vi "Main Pressure Sensor.vi"() -> ()   [LabVIEW 2018]
uses:
  <vilib>/nisyscfg/Filter Mode.ctl
  <vilib>/Platform/TimedLoop/XDataNode/timing_clust.ctl
  <vilib>/Platform/TimedLoop/XDataNode/nitl_modes.ctl
  <vilib>/Platform/TimedLoop/XDataNode/wakeup.ctl
  <vilib>/DAQmx/read.llb/DAQmx Read (Analog DBL 1Chan 1Samp).vi
  <vilib>/DAQmx/write.llb/DAQmx Write (Analog DBL 1Chan 1Samp).vi
  <vilib>/DAQmx/create/scale.llb/DAQmx Create Scale (Linear).vi
  <vilib>/DAQmx/create/channels.llb/DAQmx Create Channel (AO-Voltage-Basic).vi
  <vilib>/DAQmx/create/channels.llb/DAQmx Create Channel (AI-Voltage-Basic).vi
  <vilib>/DAQmx/miscellaneous.llb/DAQmx Fill In Error Info.vi
  <vilib>/platform/TimedLoop/XDataNode/XDataNode.xnode
  <vilib>/nisyscfg/nisyscfg.lvlib
  <resource>/objmgr/nicriosae.rc
  <vilib>/Platform/TimedLoop/XDataNode/XDNodeRunTimeDep.lvlib
  <resource>/objmgr/daqmx.rc
panel:
  out "Voltage":dbl format="%0.2f"
  in  "Scale":dbl=3.0
  out "error out":errorcluster
  in  "Power":bool
  in  "dt (ms)":i64=1000
  out "Current File Size (kB)":dbl
  out "File Location":path
  in  "save":bool=TRUE
  out "Configuration Complete?":bool
  out "Acquisition Time":timestamp format="%<%H:%M:%S%2u>T"
  out "Pressure":dbl(graph)
  # "The code will take the input voltage and\nscale it according to the Scale value to the\nright.  The measurement is set for 0-5 V, so\nif the range of the transducer is 0-15 PSI, \nthe scale should be 3; if 0-50 PSI, it should \nbe 10.\nThe system will convert PSI to inHg using \nthe conversion of 2.03602045718904 inHg \nto 1 PSI.\nTo get the maximum resolution of the \nmeasurement, divide 10 V by the \ncard resolution (2^16 if 16 bits, 2^24 if \n24 bits).  This will give you a resolution in\nV."
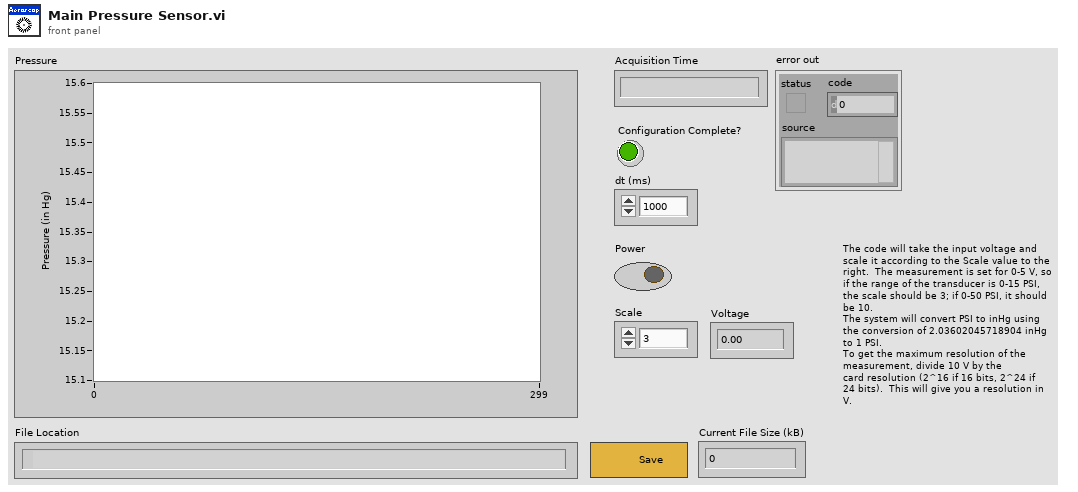
[diagram p1: front panel]
types:
  T1 = typedef "nisyscfg.lvlib/Filter Mode.ctl" = i32
  T2 = cluster{"seconds since 1Jan1904":timestamp, "data":dbl, "data 2":dbl}
  T3 = typedef "XDNodeRunTimeDep.lvlib/timing_clust.ctl" = cluster{"Expected End [f-1]":u64, "Actual End [f-1]":u64, "Finished Late? [f-1]":bool, "Expected End [i-1]":u64, "Actual End [i-1]":u64, "Finished Late? [i-1]":bool, "Expected Start [i]":u64, "Actual Start [i]":u64, "Expected Start [f]":u64, "Actual Start [f]":u64, "Source Name":string, "Structure Name":string, "Period":i64, "Deadline":i64, "Offset":i64, "Start":i64, "Priority":i32, "Timeout":i32, "Mode":T4, "Wakeup Reason":T5, "Error":errorcluster, "Source Type":string, "Secondary Source Type":string, "Global End Time":u64, "Global Start Time":u64, "Frame Duration":u64, "Iteration Duration":u64, "Assigned CPU":i32, "I/O Scan Engine Mode":u32}
  T4 = typedef "XDNodeRunTimeDep.lvlib/nitl_modes.ctl" = enum32{"No Change", "Process missed periods, maintain original phase", "Discard missed periods, maintain original phase", "Process missed periods, ignore original phase", "Discard missed periods, ignore original phase"}
  T5 = typedef "XDNodeRunTimeDep.lvlib/wakeup.ctl" = enum32{"Normal", "Aborted", "Asynchronous wakeup", "Timing source error", "Timed loop error", "Timeout"}
  T6 = cluster{"seconds since 1Jan1904":timestamp, "data":dbl, dbl}
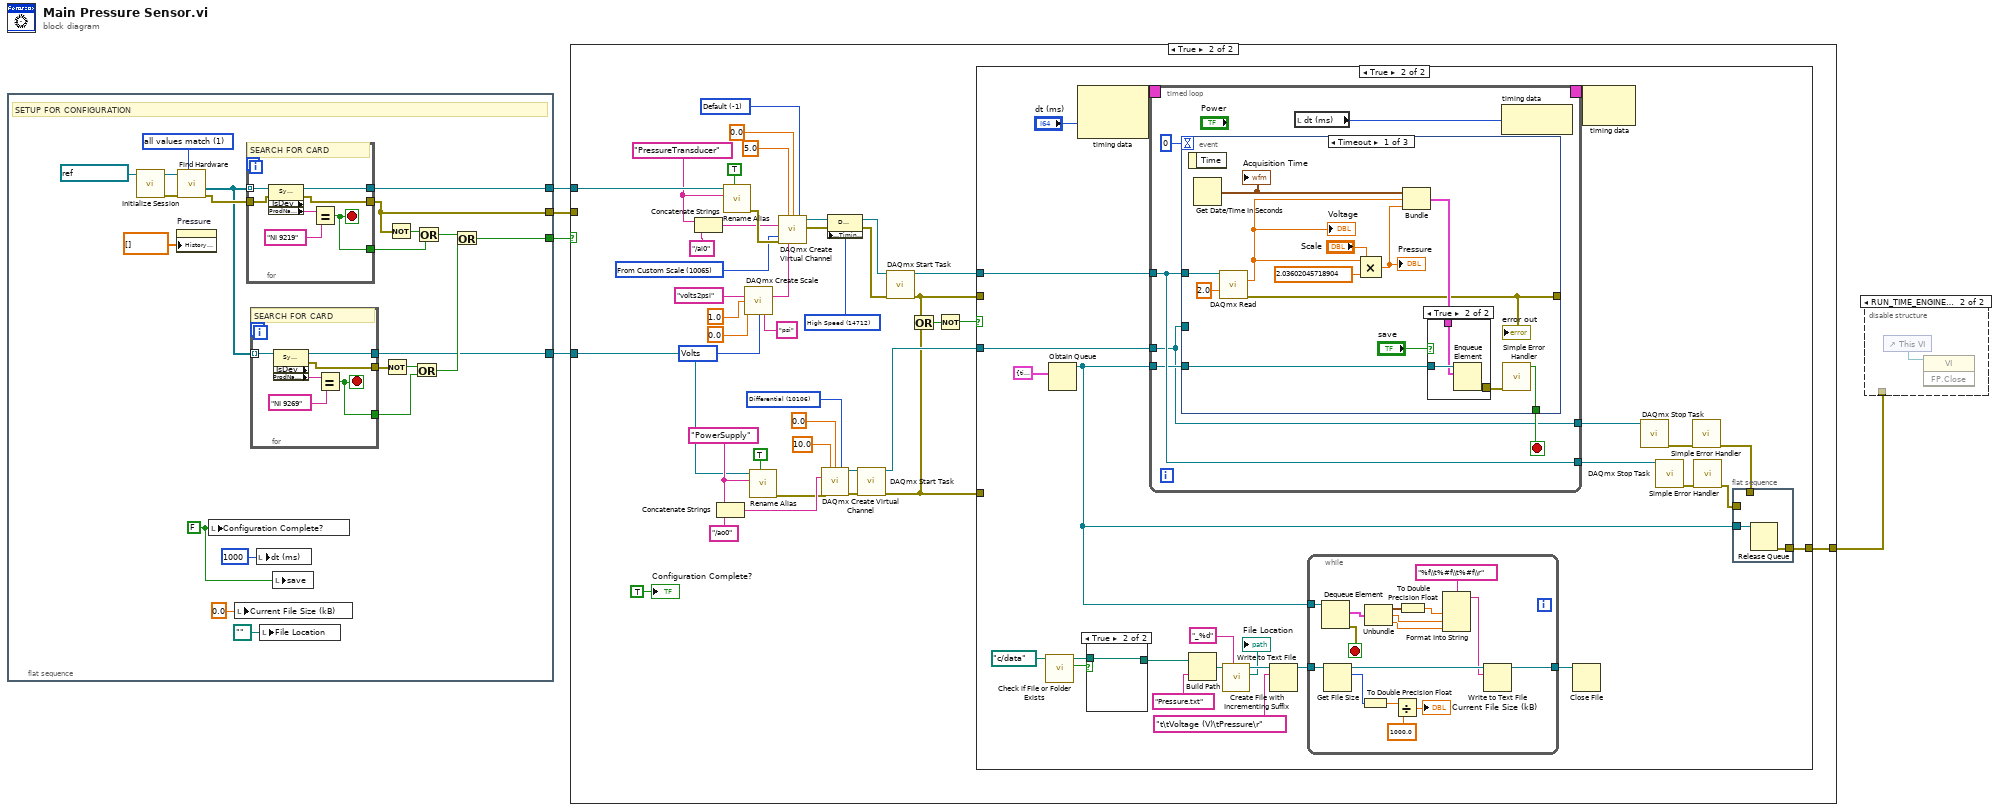
[diagram p0: block diagram]
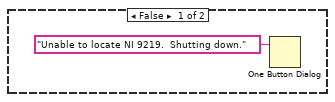
[diagram p3: hidden frame]
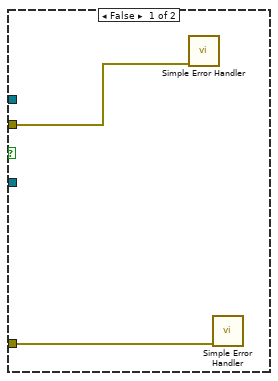
[diagram p4: hidden frame]
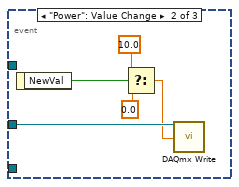
[diagram p6: hidden frame]
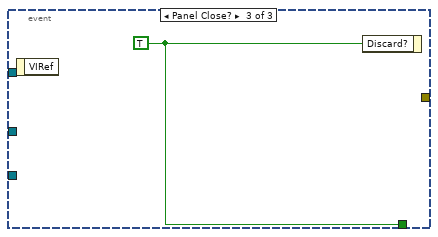
[diagram p7: hidden frame]
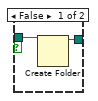
[diagram p8: hidden frame]
diagram:
  n1 = flat-sequence {
    tunnel: [w23] -> w5
    tunnel: [w20] -> w4
    tunnel: [w7] -> w3
    tunnel: [w6] -> w1
    frame #0 {
      w17 = FALSE ("Configuration Complete?")
      w24 = T1 1 items=["all values match"=1, "any value matches"=2, "values do not match"=3, "all properties exist"=4] ("Filter Mode (all values match)")
      # "SETUP FOR CONFIGURATION"
      n2 = call <vilib>:"Initialize Session.vi"("Target (localhost)"=refnum<k21> "localhost") -> ("error out"=w26:errorcluster, "Session out"=w25:refnum<k21>)  [unwired: 9 in]
      n3 = property on="Pressure" class="WFChart (strict)"("History Data"=dbl[] []) -> ()  [unwired: 2 in, 2 out]
      n4 = call <vilib>:"Find Hardware.vi"("Filter Mode (all values match)"=w24, "error in (no error)"=w26, "Session in"=w25) -> ("error out"=w22:errorcluster, "Resources out"=w13:refnum<k20>[])  [unwired: 5 in, 2 out]
      n5 = local write "Configuration Complete?"(w17) -> ()
      n6 = local write "Current File Size (kB)"(0.0 ("Current File Size (kB)")) -> ()
      n7 = for {
        tunnel: w13 -> [w40] mode=indexing
        tunnel: [w38] -> w23
        tunnel: [w37] -> w21
        tunnel: w22 -> [w36]
        tunnel: [w35] -> w20
        stop <- w37 stop-if-true
        # "SEARCH FOR CARD"
        n8 = property class="System Hardware" props=["IsDev", "ProdName"](reference=w40, error in=w36) -> (reference out=w38:refnum<k20>, error out=w35:errorcluster, "ProdName"=w34:string)  [unwired: 1 out]
        n9 = Equal?(x=w34, y="NI 9219") -> (x = y?=w37:bool)
      }
      n10 = for {
        tunnel: w13 -> [w33] mode=indexing
        tunnel: [w31] -> w6
        tunnel: [w30] -> w10
        tunnel: [w29] -> w12
        stop <- w30 stop-if-true
        # "SEARCH FOR CARD"
        n11 = property class="System Hardware" props=["IsDev", "ProdName"](reference=w33) -> (reference out=w31:refnum<k20>, error out=w29:errorcluster, "ProdName"=w28:string)  [unwired: 1 in, 1 out]
        n12 = Equal?(x=w28, y="NI 9269") -> (x = y?=w30:bool)
      }
      n13 = local write "dt (ms)"(i64 1000 ("dt (ms)")) -> ()
      n14 = local write "File Location"(path "" ("File Location")) -> ()
      n15 = local write "save"(w17) -> ()
      n16 = Not(x=w12) -> (.not. x?=w11:bool)
      n17 = Not(x=w20) -> (.not. x?=w19:bool)
      n18 = Or(x=w11, y=w10) -> (x .or. y?=w9:bool)
      n19 = Or(x=w19, y=w21) -> (x .or. y?=w8:bool)
      n20 = Or(x=w8, y=w9) -> (x .or. y?=w7:bool)
    }
  }
  n21 = case shown="True" w3 {
    tunnel: w4 -> [_ _]
    tunnel: w5 -> [_ w80]
    tunnel: [_ w76] -> w2
    tunnel: w1 -> [_ w59]
    frame False {
      n22 = One Button Dialog(message="Unable to locate NI 9219.  Shutting down.") -> ()  [unwired: 1 in, 1 out]
    }
    frame True {
      w46 = 14712 items=["High Resolution"=10195, "High Speed"=14712, "Best 50 Hz Rejection"=14713, "Best 60 Hz Rejection"=14714, "Custom"=10137] ("AI.ADCTimingMode")
      w53 = 10106 items=["Default"=-1, "RSE"=10083, "Differential"=10106, "Pseudodifferential"=12529] ("output terminal configuration")
      w62 = "PowerSupply" ("New Name")
      w66 = 10348 items=["Volts"=10348, "Amps"=10342, "Deg F"=10144, "Deg C"=10143, "Deg R"=10145, "Kelvins"=10325, "Strain"=10299, "Ohms"=10384, "Hz"=10373, "Seconds"=10364, "Meters"=10219, "Inches"=10379, "Degrees"=10146, "Radians"=10273, "Ticks"=10304, "g"=10186, "m/s^2"=12470, "m/s"=15959, "in/s"=15960, "Pascals"=10081, "Newtons"=15875, "Pounds"=15876, "kgf"=15877, "psi"=15879, "bar"=15880, "Nm"=15881, "oz-in"=15882, "lb-in"=15883, "lb-ft"=15884, "Volts/Volt"=15896, "mVolts/Volt"=15897, "pCoulombs"=16103, "Coulombs"=16102, "From TEDS"=12516] ("pre-scaled units")
      w69 = 10065 items=["Volts"=10348, "From Custom Scale"=10065] ("units")
      w72 = -1 items=["Default"=-1, "RSE"=10083, "NRSE"=10078, "Differential"=10106, "Pseudodifferential"=12529] ("input terminal configuration")
      w75 = "PressureTransducer" ("New Name")
      n23 = Concatenate Strings(w75, "/ai0" ("string")) -> (w73:string)
      n24 = Concatenate Strings(w62, "/ao0" ("string")) -> (w57:string)
      n25 = call <vilib>:"Rename Alias.vi"("Update Dependencies (T)"=TRUE, "New Name"=w75, "Resource in"=w80) -> ("error out"=w74:errorcluster)  [unwired: 5 in, 3 out]
      n26 = call-poly <vilib>:"DAQmx Create Scale.vi"("name"="volts2psi", "slope"=1.0, "y-intercept"=0.0, "pre-scaled units"=w66, "scaled units"="psi") -> ("scale out"=w64:tag)  [unwired: 9 in, 1 out]
      n27 = call <vilib>:"Rename Alias.vi"("Update Dependencies (T)"=TRUE, "New Name"=w62, "Resource in"=w59) -> ("error out"=w47:errorcluster)  [unwired: 5 in, 3 out]
      n28 = call-poly <vilib>:"DAQmx Create Virtual Channel.vi"("maximum value"=5.0, "minimum value"=0.0, "input terminal configuration"=w72, "physical channels"=w73, "units"=w69, "error in"=w74, "custom scale name"=w64) -> ("task out"=w45:refnum<k21>, "error out"=w43:errorcluster)  [unwired: 7 in]
      n29 = call-poly <vilib>:"DAQmx Create Virtual Channel.vi"("maximum value"=10.0, "minimum value"=0.0, "output terminal configuration"=w53, "physical channels"=w57, "error in"=w47) -> ("task out"=w56:refnum<k21>, "error out"=w58:errorcluster)  [unwired: 9 in]
      n30 = property class="DAQmx Channel"(reference=w45, error in=w43, "Analog Input:General Properties:Digitizer/ADC:Timing Mode"=w46) -> (reference out=w44:refnum<k21>, error out=w42:errorcluster)
      n31 = call <vilib>:"DAQmx Start Task.vi"("task/channels in"=w56, "error in"=w58) -> ("task out"=w52:refnum<k21>, "error out"=w48:errorcluster)  [unwired: 12 in]
      n32 = call <vilib>:"DAQmx Start Task.vi"("task/channels in"=w44, "error in"=w42) -> ("task out"=w77:refnum<k21>, "error out"=w49:errorcluster)  [unwired: 12 in]
      n33 = Or(x=w49, y=w48) -> (x .or. y?=w51:bool)
      n34 = Not(x=w51) -> (.not. x?=w50:bool)
      n35 = case shown="True" w50 {
        tunnel: w77 -> [_ w109]
        tunnel: [_ w92] -> w76
        tunnel: w52 -> [_ w87]
        tunnel: w49 -> [w83 _]
        tunnel: w48 -> [w82 _]
        frame False {
          n36 = call <vilib>:"Simple Error Handler.vi"("error in (no error)"=w83) -> ()  [unwired: 4 in, 5 out]
          n37 = call <vilib>:"Simple Error Handler.vi"("error in (no error)"=w82) -> ()  [unwired: 4 in, 5 out]
        }
        frame True {
          n38 = call <vilib>:"Check if File or Folder Exists.vi"("path"=path "c:/data") -> ("file or folder exists?"=w103:bool, "dup path"=w102:path)  [unwired: 8 in, 1 out]
          n39 = Obtain Queue(element data type=T2 {"seconds since 1Jan1904"=timestamp(0 s since 1904-01-01), "data"=0.0, "data 2"=0.0} ("output cluster")) -> (queue out=w106:refnum<queue>)  [unwired: 4 in, 2 out]
          n40 = node-c288("dt (ms)") -> (w90:T3)  [unwired: 1 in]
          n41 = case shown="True" w103 {
            tunnel: w102 -> [w147 w148]
            tunnel: [w146 w148] -> w101
            frame False {
              n42 = Create Folder(path (use dialog)=w147) -> (created path=w146:path)  [unwired: 2 in, 2 out]
            }
            frame True {
            }
          }
          n43 = timed-loop {
            tunnel: w109 -> [w113]
            tunnel: [w113] -> w108
            tunnel: w106 -> [w112]
            timing: w90 -> [_]
            timing-out: [_] -> w89
            tunnel: w87 -> [w110]
            tunnel: [w110] -> w86
            stop <- w115 stop-if-true
            n44 = event shown="[0] Timeout" {
              selector: _ -> [_ _ _]
              dyn-events: _ -> [_ _ _]
              timeout: 0 -> [_ _ _]
              tunnel: [w131 _ w140] -> w115
              tunnel: w113 -> [w127 _ _]
              tunnel: w112 -> [w130 _ _]
              tunnel: w110 -> [_ w139 _]
              tunnel: [w124 _ _] -> _
              event Timeout {
                n45 = event-data() -> ()  [unwired: 1 in, 1 out]
                n46 = Get Date/Time In Seconds() -> (seconds since 1Jan1904=w126:timestamp)
                "Acquisition Time" <- w126
                n47 = call-poly <vilib>:"DAQmx Read.vi"("task/channels in"=w127, "timeout"=2.0) -> ("data"=w119:dbl, "error out"=w124:errorcluster)  [unwired: 11 in, 1 out]
                "error out" <- w124
                "Voltage" <- w119
                n48 = Compound Arithmetic op=MULTIPLY(w119, "Scale", 2.03602045718904 ("value")) -> (w122:dbl)
                "Pressure" <- w122
                n49 = Bundle("seconds since 1Jan1904"=w126, "data"=w119, w122) -> (w125:T6)  [unwired: 1 in]
                n50 = case shown="True" "save" {
                  tunnel: w130 -> [_ w134]
                  tunnel: [_ w133] -> w128
                  tunnel: w125 -> [_ w132]
                  frame False {
                  }
                  frame True {
                    n51 = Enqueue Element(queue=w134, element=w132) -> (error out=w133:errorcluster)  [unwired: 2 in, 2 out]
                  }
                }
                n52 = call <vilib>:"Simple Error Handler.vi"("error in (no error)"=w128) -> ("error?"=w131:bool)  [unwired: 4 in, 4 out]
              }
              event "Power": Value Change {
                n53 = event-data() -> ("NewVal"=w138:bool)  [unwired: 1 in]
                n54 = Select(t=10.0, s=w138, f=0.0) -> (s? t:f=w135:dbl)
                n55 = call-poly <vilib>:"DAQmx Write.vi"("task/channels in"=w139, "data"=w135) -> ()  [unwired: 11 in, 3 out]
              }
              event Panel Close? {
                w140 = TRUE
                n56 = event-data() -> ()  [unwired: 1 in, 1 out]
                n57 = event-data("Discard?"=w140) -> ()  [unwired: 1 in, 1 out]
              }
            }
            n58 = local read "dt (ms)"() -> (w111:i64)
            n59 = node-c288(w111) -> ()  [unwired: 1 out]
          }
          n60 = Build Path(base path=w101, name or relative path="Pressure.txt") -> (appended path=w94:path)
          n61 = call <vilib>:"Create File with Incrementing Suffix.vi"("format string (\" (%d)\")"="_%d" ("format string (\" (%d)\")"), "file path"=w94) -> ("actual path"=→"File Location":path, "refnum out"=w96:refnum<file>)  [unwired: 7 in, 1 out]
          n62 = Write to Text File(file (use dialog)=w96, text="t\tVoltage (V)\tPressure\r") -> (refnum out=w95:refnum<file>)  [unwired: 2 in, 2 out]
          n63 = while {
            tunnel: w106 -> [w166]
            tunnel: w95 -> [w161]
            tunnel: [w164] -> w98
            stop <- w165 stop-if-true
            n64 = Dequeue Element(queue=w166) -> (element=w157:T2, error out=w165:errorcluster)  [unwired: 2 in, 2 out]
            n65 = Get File Size(file=w161) -> (refnum out=w160:refnum<file>, size (in bytes)=w159:i64)  [unwired: 1 in, 1 out]
            n66 = To Double Precision Float(number=w159) -> (double precision float=w158:dbl)
            n67 = Unbundle(w157) -> ("seconds since 1Jan1904"=w156:timestamp, "data"=w153:dbl, "data 2"=w151:dbl)
            n68 = Divide(x=w158, y=1000.0) -> (x/y=→"Current File Size (kB)":dbl)
            n69 = To Double Precision Float(number=w156) -> (double precision float=w154:dbl)
            n70 = Format Into String(format string="%f\\t%#f\\t%#f\\r", w154, w153, w151) -> (resulting string=w152:string)  [unwired: 2 in, 1 out]
            n71 = Write to Text File(file (use dialog)=w160, text=w152) -> (refnum out=w164:refnum<file>)  [unwired: 2 in, 2 out]
          }
          n72 = Close File(refnum=w98) -> ()  [unwired: 1 in, 2 out]
          n73 = node-c288(w89) -> ()  [unwired: 1 out]
          n74 = call <vilib>:"DAQmx Stop Task.vi"("task/channels in"=w86) -> ("error out"=w85:errorcluster)  [unwired: 13 in, 1 out]
          n75 = call <vilib>:"DAQmx Stop Task.vi"("task/channels in"=w108) -> ("error out"=w107:errorcluster)  [unwired: 13 in, 1 out]
          n76 = call <vilib>:"Simple Error Handler.vi"("error in (no error)"=w85) -> ("error out"=w84:errorcluster)  [unwired: 4 in, 4 out]
          n77 = call <vilib>:"Simple Error Handler.vi"("error in (no error)"=w107) -> ("error out"=w105:errorcluster)  [unwired: 4 in, 4 out]
          n78 = flat-sequence {
            tunnel: w106 -> [w150]
            tunnel: w105 -> [_]
            tunnel: [w149] -> w92
            tunnel: w84 -> [_]
            frame #0 {
              n79 = Release Queue(queue=w150) -> (error out=w149:errorcluster)  [unwired: 2 in, 2 out]
            }
          }
        }
      }
      "Configuration Complete?" <- TRUE ("Configuration Complete?")
    }
  }
  n80 = disable-structure shown="RUN_TIME_ENGINE==True" {
    disable-tunnel: w2 -> [_ _]
    frame condition #0 (active) {
    }
    frame condition #1 {
      n81 = control-ref of="This VI"() -> (w167:refnum<vi>)
      n82 = invoke class="VI" method="FP.Close"(reference=w167) -> ()  [unwired: 2 in, 3 out]
    }
  }
